vi "Process-error.vi"(8 "error in (no error)":errorcluster, 11 "Client in":T1) -> (0 "error out":errorcluster, 3 "Client out":T1)   [LabVIEW 2013, in "PowderDeposition.lvlib" / "PD-Client.lvclass"]
doc: "Processes any previously encountered error.\nThis function can process both the standard LabVIEW errors and the custom defined errors for this module.\nThe default implementation simply shows an error message box to the user and removes the error from the stream, without further affecting the program execution."
uses:
  PD-Client.lvclass
  Object-reference.ctl
  <vilib>/Utility/error.llb/DialogType.ctl
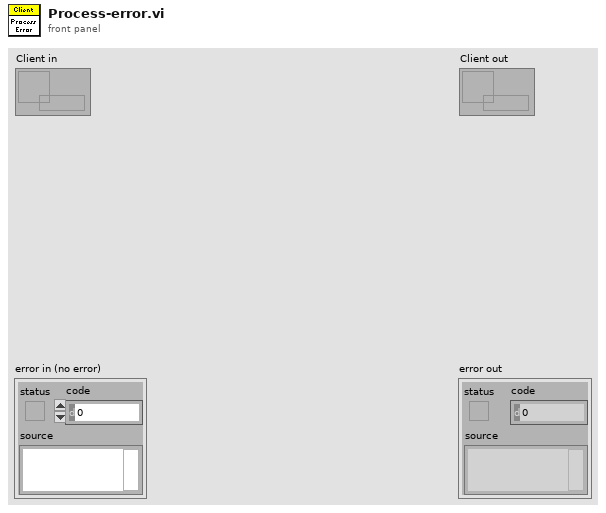
[diagram p1: front panel]
types:
  T1 = typedef "PowderDeposition.lvlib/PD-Client.lvclass/Object-reference.ctl" = refnum<data-value>
  T2 = typedef "DialogType.ctl" = u16
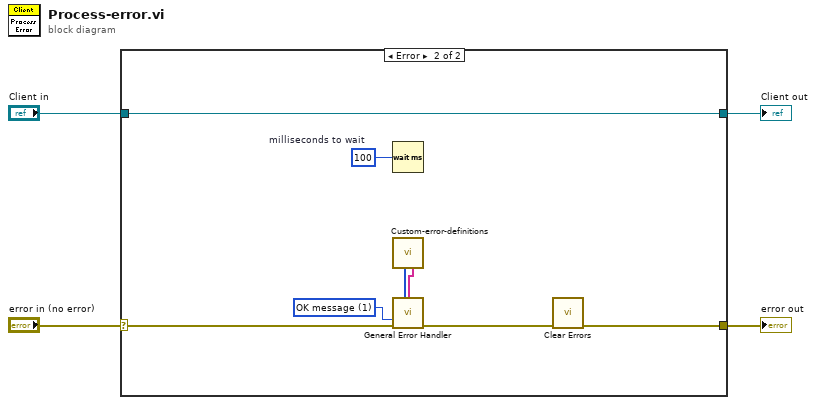
[diagram p0: block diagram]
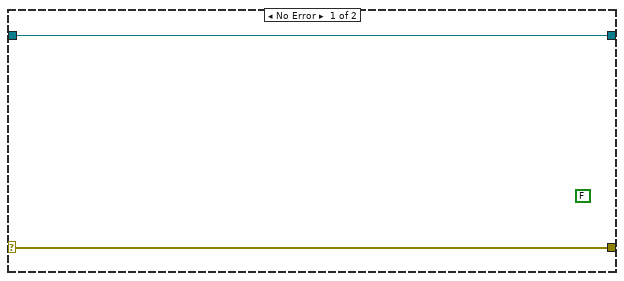
[diagram p2: hidden frame]
diagram:
  n1 = case shown="Error" "error in (no error)" {
    selector: "error in (no error)" -> [w6 w10]
    tunnel: [w6 w12] -> w3
    tunnel: [w5 w14] -> w1
    tunnel: "Client in" -> [w5 w14]
    frame No Error {
      (unwired) FALSE
    }
    frame Error {
      w7 = T2 1 items=["no dialog", "OK message", "continue or stop message", "OK message + warnings", "continue/stop + warnings"] ("type of dialog (OK msg:1)")
      w11 = u32 100  # milliseconds to wait
      n2 = Wait (ms)(milliseconds to wait=w11) -> ()  [unwired: 1 out]
      n3 = call "Custom-error-definitions.vi"() -> ("Descriptions"=w8:string[], "Error codes"=w9:i32[])  [unwired: 9 in, 1 out]
      n4 = call <vilib>:"General Error Handler.vi"("[user-defined codes]"=w9, "[user-defined descriptions]"=w8, "type of dialog (OK msg:1)"=w7, "error in (no error)"=w10) -> ("error out"=w13:errorcluster)  [unwired: 7 in, 4 out]
      n5 = call <vilib>:"Clear Errors.vi"("error in (no error)"=w13) -> ("error out"=w12:errorcluster)  [unwired: 6 in]
    }
  }
  "error out" <- w3
  "Client out" <- w1
